vi "manage Buffer.vi"(0 "Cluster":T2, 2 "Buffer in":T1(array[cluster]), 3 "Main Index":u64, 4 "Analysis Buffersize":i32) -> (5 "Buffer out":T1(array[cluster]))   [LabVIEW 2009]
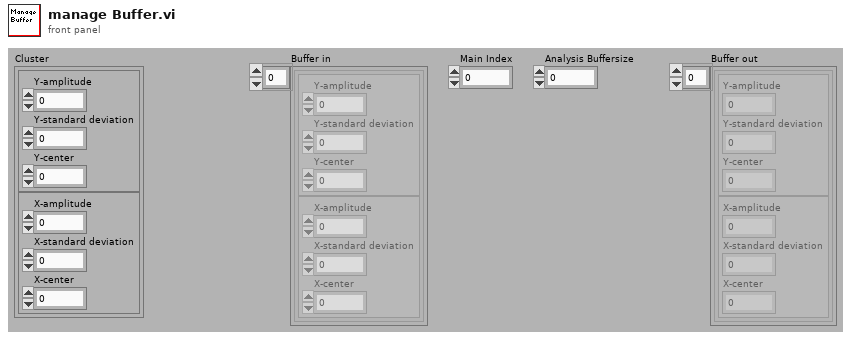
[diagram p1: front panel]
types:
  T1 = cluster{cluster{"Y-amplitude":dbl, "Y-standard deviation":dbl, "Y-center":dbl}, cluster{"X-amplitude":dbl, "X-standard deviation":dbl, "X-center":dbl}}[]
  T2 = cluster{cluster{"Y-amplitude":dbl, "Y-standard deviation":dbl, "Y-center":dbl}, cluster{"X-amplitude":dbl, "X-standard deviation":dbl, "X-center":dbl}}
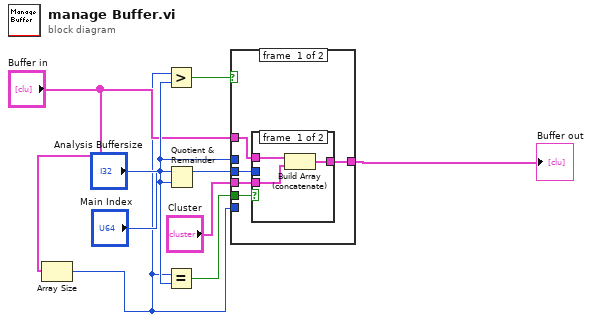
[diagram p0: block diagram]
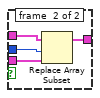
[diagram p2: hidden frame]
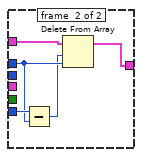
[diagram p3: hidden frame]
diagram:
  n1 = Array Size(array="Buffer in") -> (size(s)=w1:i32)
  n2 = Greater?(x=w1, y="Analysis Buffersize") -> (0:w3:bool)
  n3 = Equal?(x=w1, y="Analysis Buffersize") -> (x = y?=w9:bool)
  n4 = Quotient & Remainder(x="Main Index", y="Analysis Buffersize") -> (x-y*floor(x/y)=w6:u64)  [unwired: 1 out]
  n5 = case shown="False" w3 {
    tunnel: [w10 w22] -> w7
    tunnel: "Buffer in" -> [w11 w26]
    tunnel: "Analysis Buffersize" -> [_ w24]
    tunnel: w1 -> [_ w25]
    tunnel: "Cluster" -> [w12 _]
    tunnel: w6 -> [w13 _]
    tunnel: w9 -> [w14 _]
    frame #0 {
      n6 = case shown="True" w14 {
        tunnel: w13 -> [_ w21]
        tunnel: w12 -> [w16 w20]
        tunnel: w11 -> [w17 w19]
        tunnel: [w15 w18] -> w10
        frame #0 {
          n7 = Build Array (concatenate)(w17, w16) -> (w15:T1)
        }
        frame #1 {
          n8 = Replace Array Subset(array=w19, new element=w20, index=w21) -> (w18:T1)
        }
      }
    }
    frame #1 {
      n9 = Subtract(x=w25, y=w24) -> (x-y=w23:i32)
      n10 = Delete From Array(array=w26, length=w23, index=w24) -> (array with subset deleted=w22:T1)  [unwired: 1 out]
    }
  }
  "Buffer out" <- w7
